vi "FestoCPX.Station.ProdSuctionGripper.Clear.vi"(8 "error in":errorcluster) -> (0 "error out":errorcluster, 2 "States before clear":bool[](array[boolean]))   [LabVIEW 2016]
uses:
  FestoCPX.DO.Signal.ctl
  Station/Station.ProductSuctionGripper.Type.ctl
  Station/Station.ValvePosition.ctl
  FestoCPX.DO.Data.States.Clear.vi
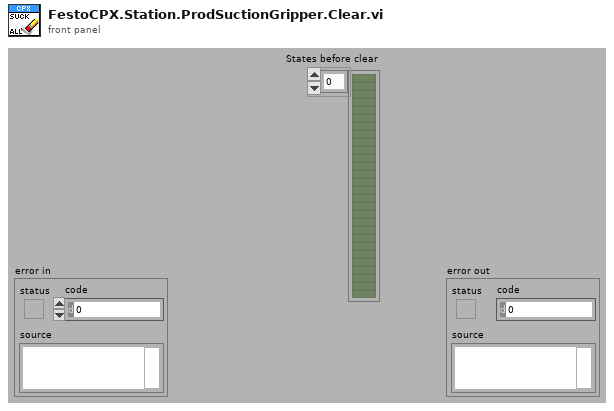
[diagram p1: front panel]
types:
  T1 = typedef "FestoCPX.DO.Signal.ctl" = enum16{"Safety Reset", "Air Main Valve", "Door Lock", "Button LED Start", "Button LED Stop", "Button LED Control", "Traffic LED Red", "Traffic LED Orange", "Traffic LED Green", "Horn", "Laser Interlock", "Laser Trigger", "Laser Fume Extractor", "Product Suction Gripper Slot 1 A", "Product Suction Gripper Slot 1 B", "Product Suction Gripper Slot 2 A", "Product Suction Gripper Slot 2 B", "Product Suction Gripper Slot 3 A", "Product Suction Gripper Slot 3 B", "Product Suction Gripper Slot 4 A", "Product Suction Gripper Slot 4 B", "Product Suction Gripper Final A", "Product Suction Gripper Final B", "Lamp", "Q1 Product Move Work", "Q1 Product Move Home", "Q2 Table Turn Work", "Q2 Table Turn Home", "Q3 Product Lift A", "Q3 Product Lift B", "Q4 Product Arm OK", "Q4 Product Arm NOK", "Q5 Product Arm Work", "Q6 Product BlowOut A", "Q6 Product BlowOut B"}
  T2 = typedef "Station.ValvePosition.ctl" = enum16{"Home", "Work"}
  T3 = typedef "Station.ProductSuctionGripper.Type.ctl" = enum8{"Final A", "Final B", "Slot 1 A", "Slot 1 B", "Slot 2 A", "Slot 2 B", "Slot 3 A", "Slot 3 B", "Slot 4 A", "Slot 4 B"}
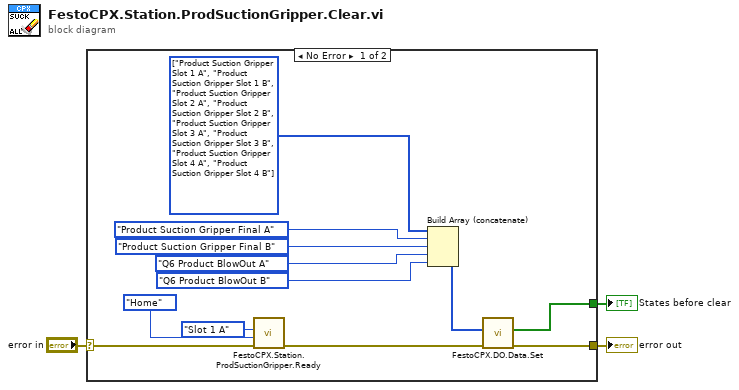
[diagram p0: block diagram]
diagram:
  n1 = case shown="No Error" "error in" {
    selector: "error in" -> [w14 w16]
    tunnel: [w15 w16] -> w3
    tunnel: [w7 _] -> w1
    frame No Error {
      w6 = T1[] [enum."Product Suction Gripper Slot 1 A", enum."Product Suction Gripper Slot 1 B", enum."Product Suction Gripper Slot 2 A", enum."Product Suction Gripper Slot 2 B", enum."Product Suction Gripper Slot 3 A", enum."Product Suction Gripper Slot 3 B", enum."Product Suction Gripper Slot 4 A", enum."Product Suction Gripper Slot 4 B"] items=["Safety Reset", "Air Main Valve", "Door Lock", "Button LED Start", "Button LED Stop", "Button LED Control", "Traffic LED Red", "Traffic LED Orange", "Traffic LED Green", "Horn", "Laser Interlock", "Laser Trigger", "Laser Fume Extractor", "Product Suction Gripper Slot 1 A", "Product Suction Gripper Slot 1 B", "Product Suction Gripper Slot 2 A", "Product Suction Gripper Slot 2 B", "Product Suction Gripper Slot 3 A", "Product Suction Gripper Slot 3 B", "Product Suction Gripper Slot 4 A", "Product Suction Gripper Slot 4 B", "Product Suction Gripper Final A", "Product Suction Gripper Final B", "Lamp", "Q1 Product Move Work", "Q1 Product Move Home", "Q2 Table Turn Work", "Q2 Table Turn Home", "Q3 Product Lift A", "Q3 Product Lift B", "Q4 Product Arm OK", "Q4 Product Arm NOK", "Q5 Product Arm Work", "Q6 Product BlowOut A", "Q6 Product BlowOut B"] ("CPX.DO")
      n2 = call "FestoCPX.Station.ProdSuctionGripper.Ready.vi"("error in"=w14, "Position"=Station.ValvePosition."Home", "Type"=Station.ProductSuctionGripper.Type."Slot 1 A") -> ("error out"=w13:errorcluster)  [unwired: 7 in, 1 out]
      n3 = Build Array (concatenate)(w6, FestoCPX.DO.Signal."Product Suction Gripper Final A" ("CPX.DO"), FestoCPX.DO.Signal."Product Suction Gripper Final B" ("CPX.DO"), FestoCPX.DO.Signal."Q6 Product BlowOut A" ("CPX.DO"), FestoCPX.DO.Signal."Q6 Product BlowOut B" ("CPX.DO")) -> (w9:T1[])
      n4 = call-poly "FestoCPX.DO.Data.Set.vi"("error in (no error)"=w13, "CPX.DO"=w9) -> ("error out"=w15:errorcluster, "States before clear"=w7:bool[])  [unwired: 8 in]
    }
    frame Error {
    }
  }
  "error out" <- w3
  "States before clear" <- w1
